vi "CRYPlot Digital Graph.vi"(7 "pGraph VI In":refnum<vi>, 11 "Selected Row In":i32[](array[numeric])) -> (1 "Color Info":u32[](array[numeric]), 2 "Curve Name":string[](array[string]), 3 "Selected Row Out":i32[](array[numeric]))   [LabVIEW 2013]
uses:
  <vilib>/Waveform/DWDTOps.llb/Digital Pattern Generator (Random).vi
panel:
  out "Signal Number":i32
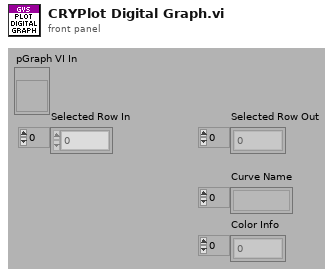
[diagram p1: front panel]
types:
  T1 = typedef "CRYData Cluster.ctl" = cluster{"Name":string, "Curve":cluster{"x":dbl, "y":dbl, "z":dbl}[], "X data":u16, "Y data":u16, "Z data":u16, "X axis":u16, "Y axis":u16, "Z axis":u16, "X unit":string, "Y unit":string, "Z unit":string, "X dB ref":dbl, "Y dB ref":dbl, "Z dB ref":dbl, "single val":bool, "protected":bool, "display X":bool, "display Y":bool, "display Z":bool, "Test Info":string, "Step No.":i32, "Plot Settings":cluster{"Color":u32, "Interpolation":u8, "Point Style":u8, "Line Style":u8, "Point Color":u32, "Line Width":u8, "Bar Plot Style":u8, "Fill To":i16}, "AutoProtect":bool}
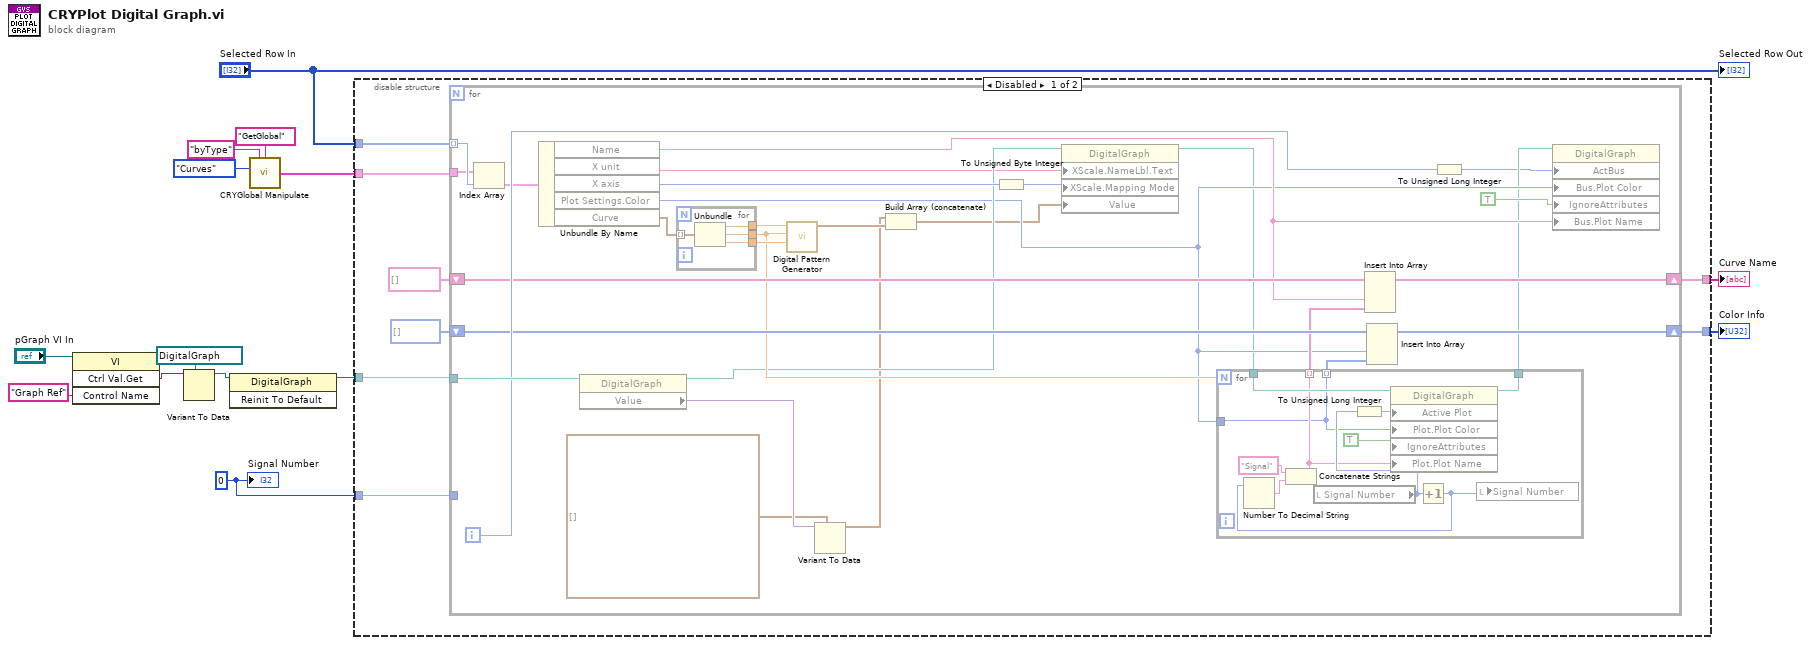
[diagram p0: block diagram]
diagram:
  w10 = 0 ("Numeric")
  n1 = invoke class="VI" method="Ctrl Val.Get"(reference="pGraph VI In", "Control Name"="Graph Ref") -> ("Get Control Value Variant"=w8:variant)  [unwired: 2 in, 3 out]
  n2 = Variant To Data(type=refnum<vi> refnum ("Graph Ref"), Variant=w8) -> (data=w5:refnum<vi>)  [unwired: 1 in, 1 out]
  n3 = invoke class="DigitalGraph" method="Reinit To Default"(reference=w5) -> (reference out=w14:refnum<vi>)  [unwired: 2 in, 2 out]
  n4 = call "CRYGlobal Manipulate.vi"("Type"=enum16{"Curves", "Values", "Results", "WFM"}."Curves", "sOption"="byType", "sAction"="GetGlobal") -> ("Curves Out"=w1:T1[])  [unwired: 6 in, 6 out]
  n5 = disable-structure shown="Disabled" {
    disable-tunnel: w14 -> [w22 _]
    disable-tunnel: "Selected Row In" -> [w19 _]
    disable-tunnel: [w18 _] -> w12
    disable-tunnel: [w17 _] -> w11
    disable-tunnel: w10 -> [w16 _]
    disable-tunnel: w1 -> [w15 _]
    frame Disabled {
      n6 = for {
        tunnel: w22 -> [w50]
        tunnel: w19 -> [w51] mode=indexing
        tunnel: w15 -> [w49]
        shift-right: [w47] -> w18
        shift-left: string[] [] -> [w46]
        shift-right: [w45] -> w17
        shift-left: u32[] [] -> [w44]
        tunnel: w16 -> [_]
        i -> [w48]
        n7 = Index Array(array=w49, index=w51) -> (element=w38:T1)
        n8 = Unbundle By Name(w38) -> ("Name"=w33:string, "X unit"=w34:string, "X axis"=w52:u16, "Plot Settings.Color"=w32:u32, "Curve"=w42:cluster{"x":dbl, "y":dbl, "z":dbl}[])
        n9 = property class="DigitalGraph"(reference=w50) -> (reference out=w37:refnum<vi>, "Value"=w28:variant)  [unwired: 1 in, 1 out]
        n10 = for {
          tunnel: w42 -> [w56] mode=indexing
          tunnel: [w55] -> w41
          tunnel: [w54] -> w39
          tunnel: [w53] -> w40
          n11 = Unbundle(w56) -> ("x"=w55:dbl, "y"=w54:dbl, "z"=w53:dbl)
        }
        n12 = call-poly <vilib>:"Digital Pattern Generator.vi"("sample rate"=w40, "number of signals"=w39, "number of samples"=w41) -> ("digital waveform"=w29:digitalwaveform)  [unwired: 1 in, 7 out]
        n13 = Variant To Data(type=digitalwaveform[] [] ("appended array"), Variant=w28) -> (data=w27:digitalwaveform[])  [unwired: 1 in, 1 out]
        n14 = Build Array (concatenate)(w27, w29) -> (w24:digitalwaveform[])
        n15 = To Unsigned Byte Integer(number=w52) -> (unsigned 8bit integer=w26:u8)
        n16 = property class="DigitalGraph"(reference=w37, "XScale.NameLbl.Text"=w34, "XScale.Mapping Mode"=w26, "Value"=w24) -> (reference out=w31:refnum<vi>)  [unwired: 1 in, 1 out]
        n17 = for {
          N: w39 -> [_]
          tunnel: w32 -> [w60]
          tunnel: w31 -> [w64]
          tunnel: [w61] -> w36 mode=indexing
          tunnel: [w60] -> w35 mode=indexing
          tunnel: [w58] -> w30
          n18 = local read "Signal Number"() -> (w63:i32)
          n19 = To Unsigned Long Integer(number=w63) -> (unsigned 32bit integer=w57:u32)
          n20 = Increment(x=w63) -> (x+1=w62:i32)
          n21 = Number To Decimal String(number=w62) -> (decimal integer string=w66:string)  [unwired: 1 out]
          n22 = Concatenate Strings("Signal", w66) -> (w61:string)
          n23 = property class="DigitalGraph"(reference=w64, "Active Plot"=w57, "Plot.Plot Color"=w60, "IgnoreAttributes"=TRUE ("Ignore Attributes"), "Plot.Plot Name"=w61) -> (reference out=w58:refnum<vi>)  [unwired: 1 in, 1 out]
          n24 = local write "Signal Number"(w62) -> ()
        }
        n25 = Insert Into Array(array=w46, new element #1=w33, new element #2=w36) -> (w47:string[])  [unwired: 1 in]
        n26 = Insert Into Array(array=w44, new element #1=w32, new element #2=w35) -> (w45:u32[])  [unwired: 1 in]
        n27 = To Unsigned Long Integer(number=w48) -> (unsigned 32bit integer=w25:u32)
        n28 = property class="DigitalGraph"(reference=w30, "ActBus"=w25, "Bus.Plot Color"=w32, "IgnoreAttributes"=TRUE ("Ignore Attributes"), "Bus.Plot Name"=w33) -> ()  [unwired: 1 in, 2 out]
      }
    }
    frame Enabled {
    }
  }
  "Curve Name" <- w12
  "Color Info" <- w11
  "Signal Number" <- w10
  "Selected Row Out" <- "Selected Row In"
